vi "In_S2F37.vi"(8 "error in (no error)":errorcluster, 11 "S2 Message Class in":refnum<class "S2 Message Class.lvclass">) -> (0 "error out":errorcluster, 1 "OK?":bool, 2 "S2F37":T1, 3 "S2 Message Class out":refnum<class "S2 Message Class.lvclass">)   [LabVIEW 2020, in "SECS Communication.lvlib" / "S2 Message Class.lvclass"]
uses:
  S2 Message Class.lvclass
  D:/Dropbox/SECS/SECS_GEM v1.0.7/Com/SECS Communication/SECS-II Class/SECS-II Class.lvclass
  S2F37.ctl
  SECS-II Class/SECS-II Class.lvclass/SECS-II Class.ctl
  SECS-II Class/Variant To Data_Boolean.vi
  SECS-II Class/Variant To Data_U4.vi
  SECS-II Class/SECS-II Class.lvclass
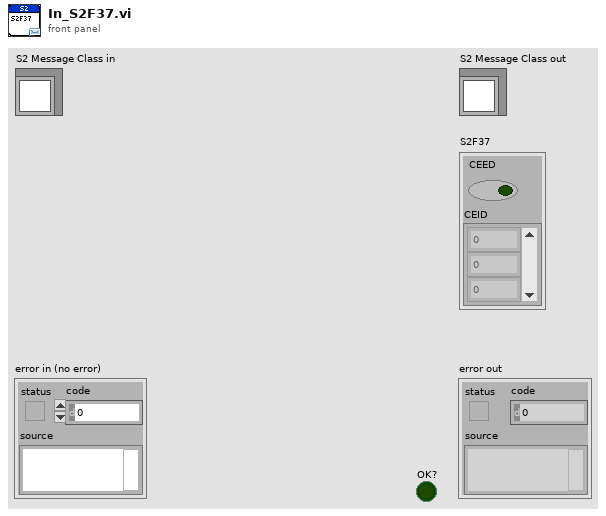
[diagram p1: front panel]
types:
  T1 = typedef "SECS Communication.lvlib/S2 Message Class.lvclass/S2F37.ctl" = cluster{"CEED":bool, "CEID":u32[]}
  T2 = typedef "SECS Communication.lvlib/SECS-II Class.lvclass/Message Data.ctl" = cluster{"Index":i32, "Data Item Format":T3, "Format Code":T4, "Parent Index":i32, "Child Index":i32[], "Data":variant}
  T3 = typedef "SECS Communication.lvlib/SECS-II Class.lvclass/Data Item Format.ctl" = enum16{"Data Type", "Value"}
  T4 = typedef "SECS Communication.lvlib/SECS-II Class.lvclass/Format Code.ctl" = enum16{"L", "A", "B", "Boolean", "J", "I1", "I2", "I4", "I8", "U1", "U2", "U4", "U8", "F4", "F8", "Char"}
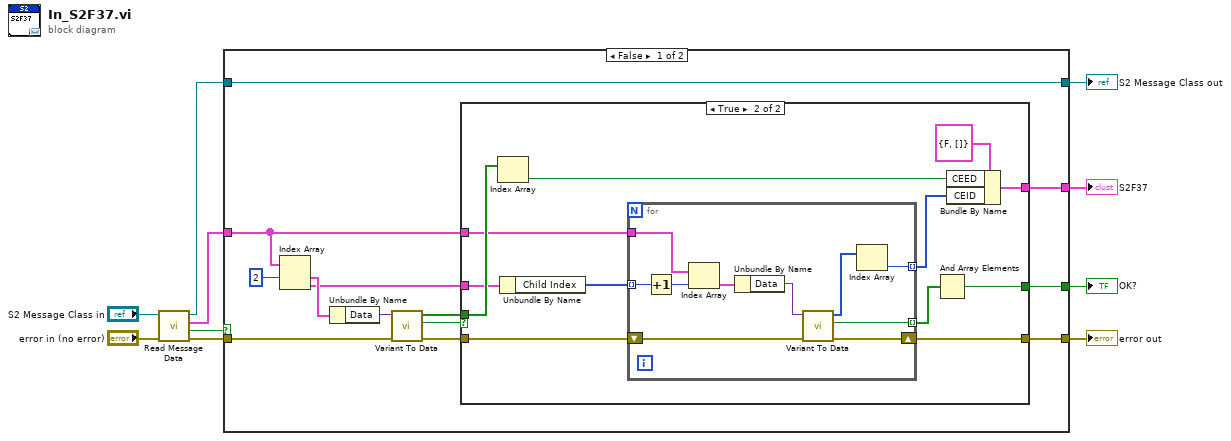
[diagram p0: block diagram]
diagram:
  n1 = call "Read Message Data.vi"("error in (no error)"="error in (no error)", "SECS-II Class in"="S2 Message Class in") -> ("error out"=w10:errorcluster, "Empty?"=w9:bool, "Message Data"=w8:T2[], "SECS-II Class out"=w7:refnum<class "S2 Message Class.lvclass">)  [unwired: 6 in]
  n2 = case shown="False" w9 {
    tunnel: w8 -> [w14 _]
    tunnel: w10 -> [w22 w47]
    tunnel: [w16 w47] -> w6
    tunnel: w7 -> [w13 w48]
    tunnel: [w13 w48] -> w1
    tunnel: [w12 _] -> w5
    tunnel: [w11 _] -> w4
    frame False {
      n3 = Index Array(array=w14, index #1=2 ("index")) -> (element #1=w21:T2, element #2=w15:T2)  [unwired: 1 in]
      n4 = Unbundle By Name(w21) -> ("Data"=w20:variant)
      n5 = call-poly "Variant To Data.vi"("error in (no error)"=w22, "Variant"=w20) -> ("error out"=w17:errorcluster, "OK?"=w18:bool, "Data"=w19:bool[])  [unwired: 7 in]
      n6 = case shown="True" w18 {
        tunnel: w19 -> [_ w36]
        tunnel: w17 -> [w24 w30]
        tunnel: [w24 w28] -> w16
        tunnel: w15 -> [_ w33]
        tunnel: w14 -> [_ w32]
        tunnel: [_ w26] -> w11
        tunnel: [_ w25] -> w12
        frame False {
        }
        frame True {
          n7 = Index Array(array=w36) -> (element=w34:bool)  [unwired: 1 in]
          n8 = Unbundle By Name(w33) -> ("Child Index"=w31:i32[])
          n9 = for {
            tunnel: w32 -> [w45]
            tunnel: w31 -> [w46] mode=indexing
            shift-right: [w40] -> w28
            shift-left: w30 -> [w42]
            tunnel: [w38] -> w29 mode=indexing
            tunnel: [w37] -> w27 mode=indexing
            n10 = Increment(x=w46) -> (x+1=w44:i32)
            n11 = Index Array(array=w45, index=w44) -> (element=w43:T2)
            n12 = Unbundle By Name(w43) -> ("Data"=w41:variant)
            n13 = call-poly "Variant To Data.vi"("error in (no error)"=w42, "Variant"=w41) -> ("error out"=w40:errorcluster, "OK?"=w37:bool, "Data"=w39:u32[])  [unwired: 7 in]
            n14 = Index Array(array=w39) -> (element=w38:u32)  [unwired: 1 in]
          }
          n15 = And Array Elements(Boolean array=w27) -> (logical AND=w26:bool)
          n16 = Bundle By Name(cluster=T1 {"CEED"=FALSE, "CEID"=[]} ("S2F37"), "CEED"=w34, "CEID"=w29) -> (w25:T1)
        }
      }
    }
    frame True {
    }
  }
  "error out" <- w6
  "S2 Message Class out" <- w1
  "S2F37" <- w5
  "OK?" <- w4
